vi "Popualte Names Init.vi"(8 "error in (no error)":errorcluster, 10 "Current Bus Number":i32, 11 "Destination Path":path) -> (0 "error out":errorcluster, 2 "Communication FIFOs Elements":refnum<vi>[](array[refnum]), 3 "Communication FIFOs Refnum":refnum<vi>)   [LabVIEW 2014, in "Initialization and IO Node Scripting.lvlib"]
uses:
  Initialization and IO Node Scripting.lvlib
  <vilib>/Utility/traverseref.llb/TRef TravTarget.ctl
  <vilib>/Utility/traverseref.llb/VI Scripting - Traverse.lvlib
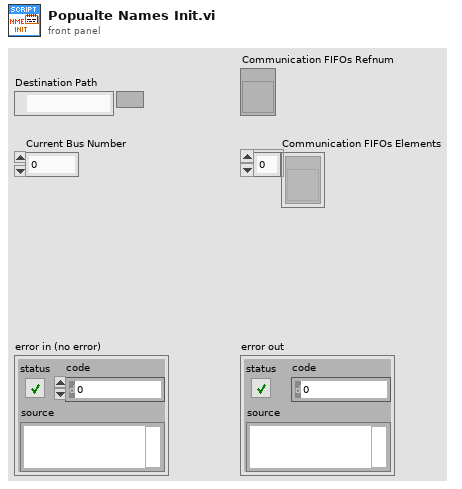
[diagram p1: front panel]
types:
  T1 = typedef "TRef TravTarget.ctl" = enum16{"FP", "BD", "Other"}
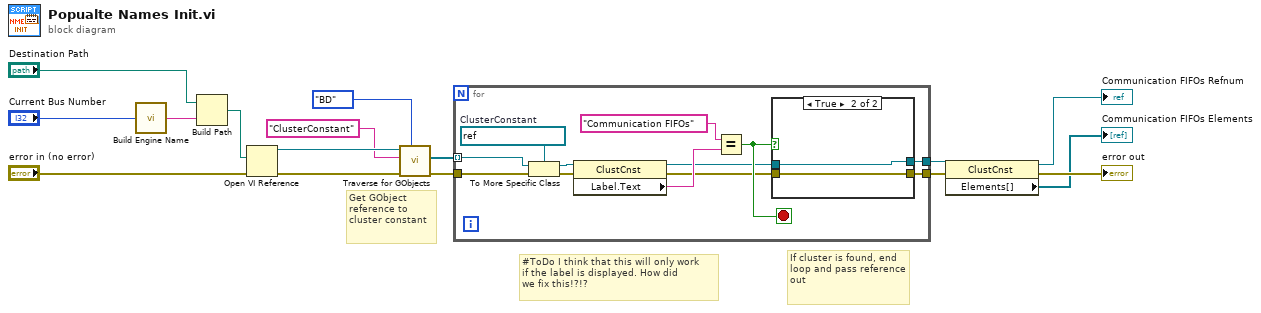
[diagram p0: block diagram]
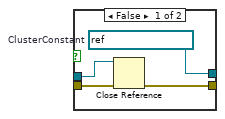
[diagram p2: hidden frame]
diagram:
  # "#ToDo I think that this will only work\nif the label is displayed. How did\nwe fix this!?!?"
  # "If cluster is found, end loop and pass reference out"
  # "Get GObject reference to cluster constant"
  n1 = call "Build Engine Name.vi"("Current Bus Number"="Current Bus Number") -> ("Engine Name"=w2:string)
  n2 = Build Path(base path="Destination Path", name or relative path=w2) -> (appended path=w9:path)
  n3 = Open VI Reference(vi path=w9, error in (no error)="error in (no error)") -> (vi reference=w12:refnum<vi>, error out=w13:errorcluster)  [unwired: 4 in]
  n4 = call <vilib>:"Traverse for GObjects.vi"("Traverse Target"=TRef_TravTarget."BD", "error in (no error)"=w13, "Class Name"="ClusterConstant", "VI Refnum"=w12) -> ("error out"=w15:errorcluster, "References"=w14:refnum<vi>[])  [unwired: 4 in, 2 out]
  n5 = for {
    tunnel: w14 -> [w26] mode=indexing
    tunnel: w15 -> [w27]
    tunnel: [w18] -> w7
    tunnel: [w17] -> w8
    stop <- w21 stop-if-true
    w28 = refnum<vi> refnum  # ClusterConstant
    n6 = To More Specific Class(target class=w28, reference=w26, error in=w27) -> (specific class reference=w24:refnum<vi>, error out=w25:errorcluster)
    n7 = property class="ClustCnst"(reference=w24, error in=w25) -> (reference out=w19:refnum<vi>, error out=w20:errorcluster, "Label.Text"=w23:string)
    n8 = Equal?(x="Communication FIFOs", y=w23) -> (x = y?=w21:bool)
    n9 = case shown="True" w21 {
      tunnel: w20 -> [w32 w34]
      tunnel: w19 -> [w31 w33]
      tunnel: [w29 w34] -> w17
      tunnel: [w30 w33] -> w18
      frame False {
        w30 = refnum<vi> refnum  # ClusterConstant
        n10 = Close Reference(reference=w31, error in (no error)=w32) -> (error out=w29:errorcluster)
      }
      frame True {
      }
    }
  }
  n11 = property class="ClustCnst"(reference=w7, error in=w8) -> (reference out=→"Communication FIFOs Refnum":refnum<vi>, error out=→"error out":errorcluster, "Elements[]"=→"Communication FIFOs Elements":refnum<vi>[])
